vi "Stop.vi"(8 "error in (no error)":errorcluster, 11 "Digital Serial in":refnum<class "Digital Serial.lvclass">) -> (0 "error out":errorcluster, 3 "Digital Serial out":refnum<class "Digital Serial.lvclass">)   [LabVIEW 2023, in "Digital Serial.lvclass"]
uses:
  Digital Serial.lvclass
  Digital Serial.lvclass/Digital Serial.ctl
  <vilib>/PDM Acquisition Toolkit/host/API/PDM Acquisition Toolkit.lvlib
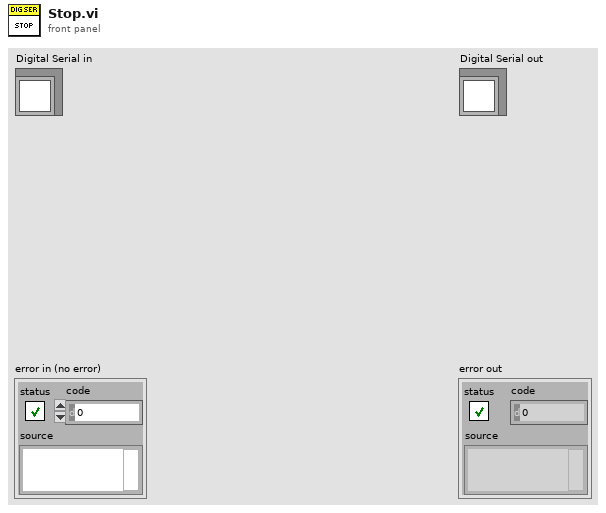
[diagram p1: front panel]
types:
  T1 = typedef "PDM Acquisition Class Library.lvlib/PCM Output Task.lvclass/PCM Output Task DVR.ctl" = refnum<data-value>
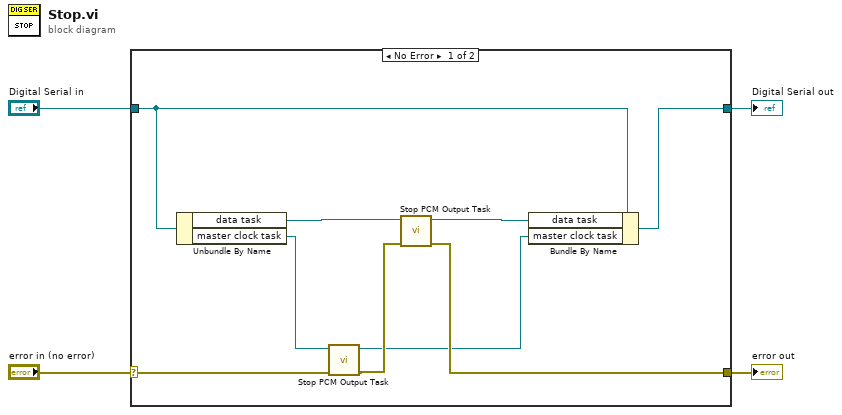
[diagram p0: block diagram]
diagram:
  n1 = case shown="No Error" "error in (no error)" {
    selector: "error in (no error)" -> [w12 w15]
    tunnel: [w11 w15] -> w3
    tunnel: [w5 w14] -> w1
    tunnel: "Digital Serial in" -> [w8 w14]
    frame No Error {
      n2 = Unbundle By Name(w8) -> ("data task"=w10:T1, "master clock task"=w9:T1)
      n3 = call <vilib>:"Stop PCM Output Task.vi"("error in"=w12, "PCM output task In"=w9) -> ("error out"=w13:errorcluster, "PCM output task out"=w6:T1)  [unwired: 8 in]
      n4 = call <vilib>:"Stop PCM Output Task.vi"("error in"=w13, "PCM output task In"=w10) -> ("error out"=w11:errorcluster, "PCM output task out"=w7:T1)  [unwired: 8 in]
      n5 = Bundle By Name(cluster=w8, "data task"=w7, "master clock task"=w6) -> (w5:refnum<class "Digital Serial.lvclass">)
    }
    frame Error {
    }
  }
  "error out" <- w3
  "Digital Serial out" <- w1
